vi "Populate SCL.vi"(8 "error in":errorcluster, 11 "SCL":refnum<vi>) -> (0 "error out":errorcluster, 2 "No Templates Found Message":string, 3 "At least one template file found?":bool)   [LabVIEW 2022 SP3]
doc: "Populates the SCL that displays the available VI templates and CTL templates, respectively.\n\nSCL = Single-Column Listbox"
uses:
  <vilib>/Utility/miscctls.llb/LVFontTypeDef.ctl
panel:
  out "All Template Filenames":string[](array[string])
  out "CTTs":string[](array[string])
  out "VITs":string[](array[string])
  out "VIs":string[](array[string])
  out "CTLs":string[](array[string])
  out "Templates Folder Location":path
  out "All Filenames In Folder":string[](array[string])
  # "Development\ncontrols/indicators useful for development and testing, but which are not outputs of the VI"
  # "Input\nInputs to the VI"
  # "Output\nOutputs of the VI"
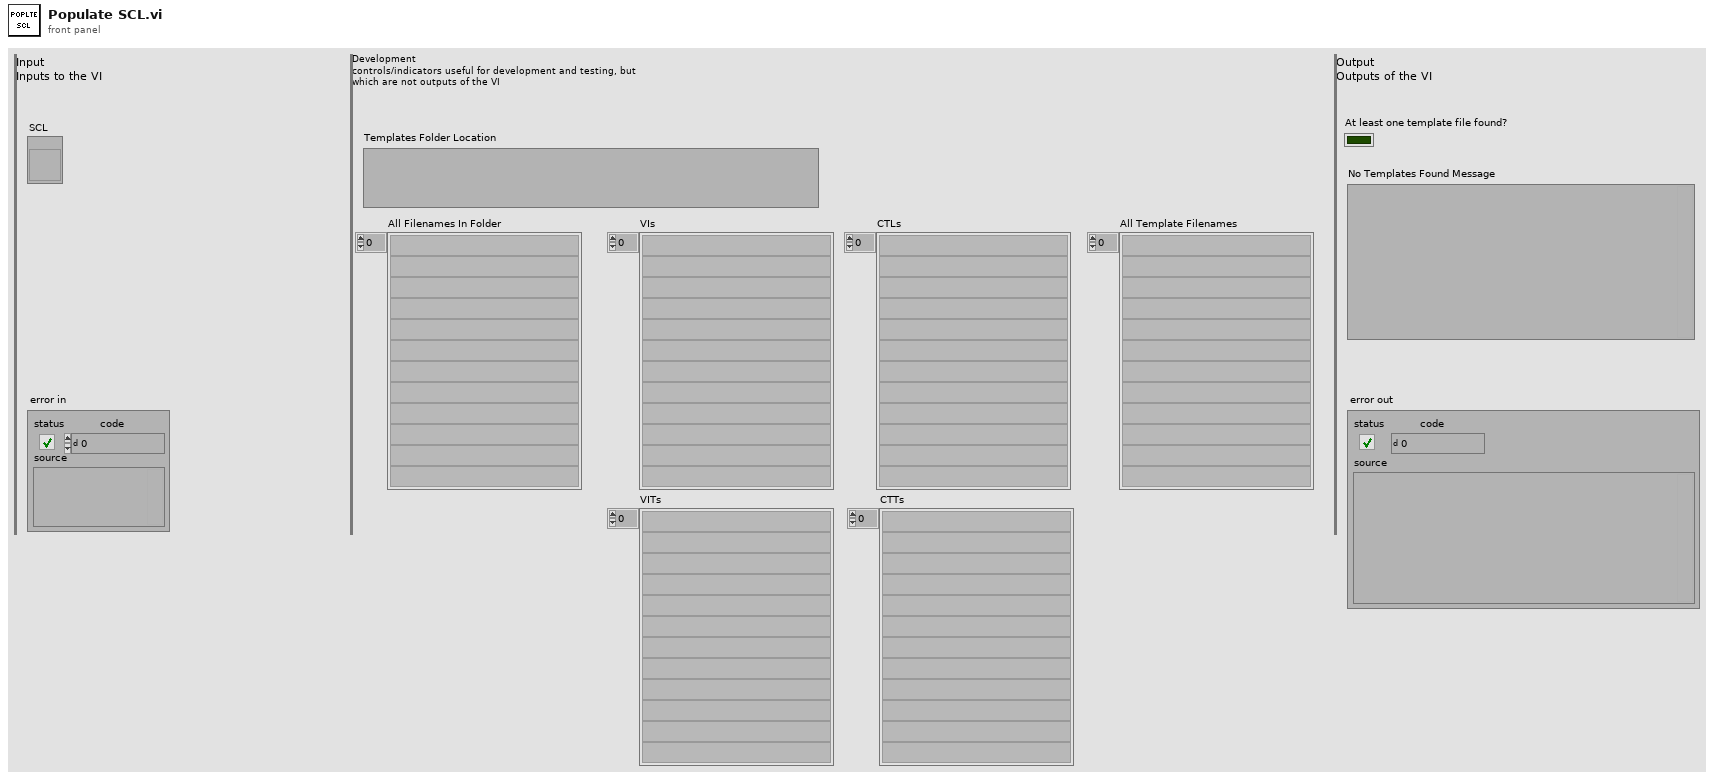
[diagram p1: front panel]
types:
  T1 = typedef "LVFontTypeDef.ctl" = cluster{"Font Name":string, "Size":u16, "Bold":bool, "Italic":bool, "Underline":bool, "Strikeout":bool, "Color":u32}
  T2 = typedef "Registry RtKey.ctl" = enum32{"HKEY_CLASSES_ROOT", "HKEY_CURRENT_USER", "HKEY_LOCAL_MACHINE", "HKEY_USERS", "HKEY_PERFORMANCE_DATA", "HKEY_CURRENT_CONFIG", "HKEY_DYN_DATA"}
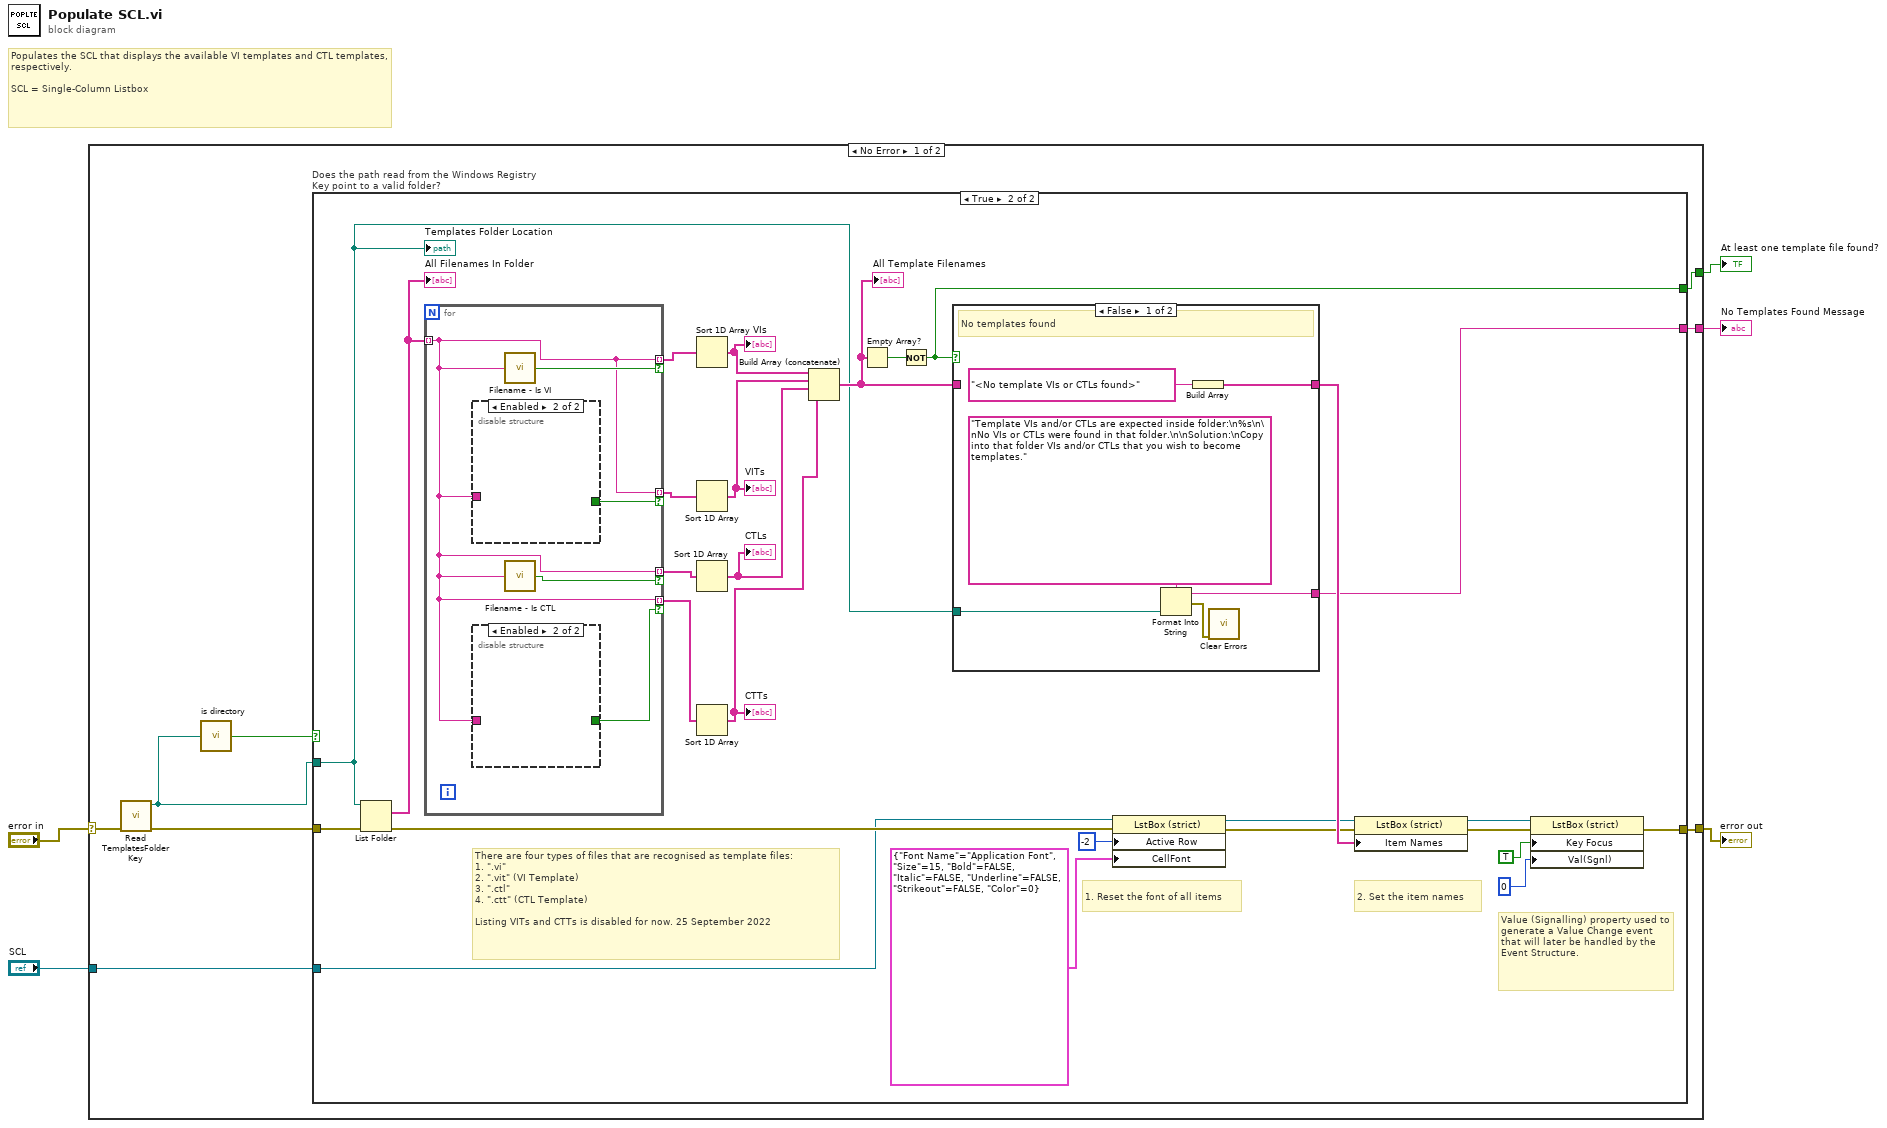
[diagram p0: block diagram]
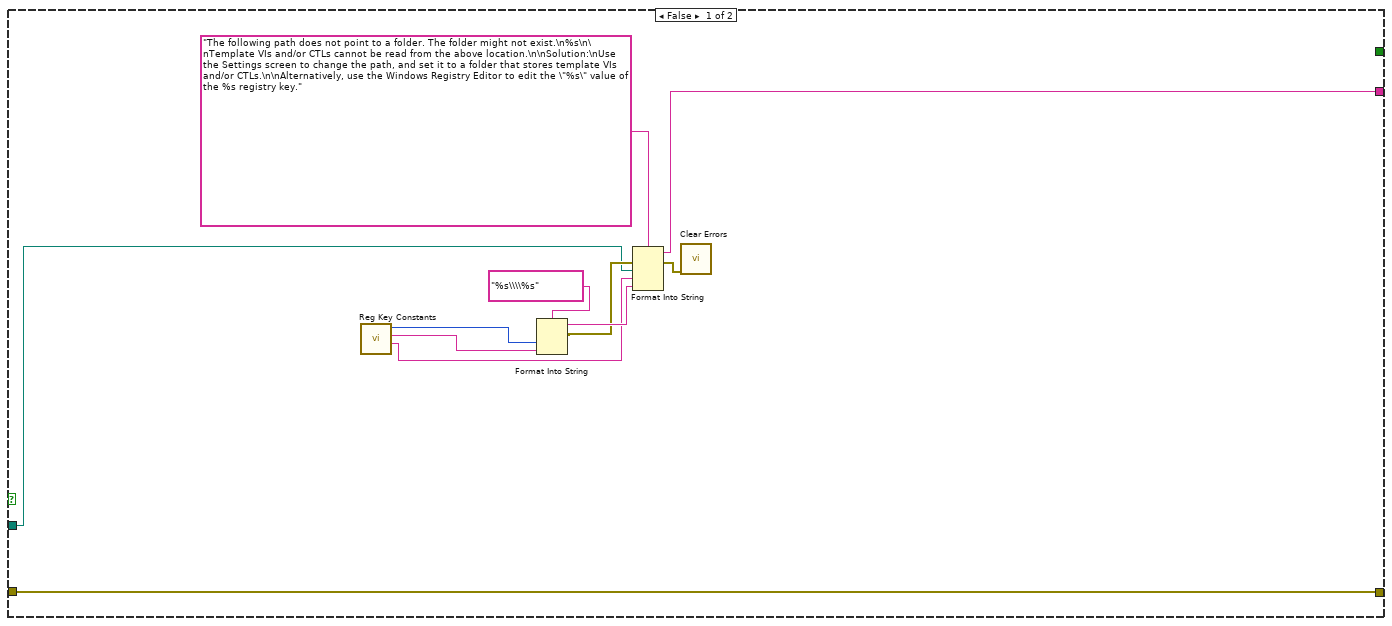
[diagram p2: hidden frame]
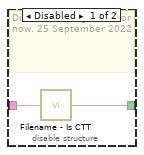
[diagram p4: hidden frame]
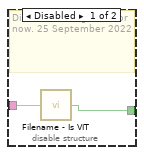
[diagram p5: hidden frame]
diagram:
  # "Populates the SCL that displays the available VI templates and CTL templates, respectively.\n\nSCL = Single-Column Listbox"
  n1 = case shown="No Error" "error in" {
    selector: "error in" -> [w10 w68]
    tunnel: [w12 w68] -> w4
    tunnel: "SCL" -> [w13 _]
    tunnel: [w11 _] -> w2
    tunnel: [w6 _] -> w1
    frame No Error {
      n2 = call "Read TemplatesFolder Key.vi"("Error In"=w10) -> ("Error Out"=w9:errorcluster, "Templates Folder Path"=w8:path)  [unwired: 9 in]
      n3 = call "is directory.vi"("Path"=w8) -> ("Does the path point to a directory (a folder)?"=w7:bool)
      n4 = case "Does the path read from the Windows Registry Key point to a valid folder?" shown="True" w7 {
        tunnel: w13 -> [_ w48]
        tunnel: [w24 w45] -> w12
        tunnel: [_ w29] -> w11
        tunnel: w9 -> [w24 w27]
        tunnel: w8 -> [w14 w26]
        tunnel: [w16 w25] -> w6
        frame False {
          n5 = call "Reg Key Constants.vi"() -> ("String Value Name"=w15:string, "Subkey Path"=w21:string, "Root Key"=w22:T2)  [unwired: 4 in, 1 out]
          n6 = Format Into String(format string="%s\\\\%s", w22, w21) -> (resulting string=w19:string, error out=w17:errorcluster)  [unwired: 2 in]
          n7 = Format Into String(format string="The following path does not point to a folder. The folder might not exist.\n%s\n\nTemplate VIs and/or CTLs cannot be read from the above location.\n\nSolution:\nUse the Settings screen to change the path, and set it to a folder that stores template VIs and/or CTLs.\n\nAlternatively, use the Windows Registry Editor to edit the \"%s\" value of the %s registry key.", error in=w17, w14, w15, w19) -> (resulting string=w16:string, error out=w18:errorcluster)  [unwired: 1 in]
          n8 = call <vilib>:"Clear Errors.vi"("error in (no error)"=w18) -> ()  [unwired: 5 in, 2 out]
        }
        frame True {
          # "Value (Signalling) property used to generate a Value Change event that will later be handled by the Event Structure."
          # "2. Set the item names"
          # "1. Reset the font of all items"
          # "There are four types of files that are recognised as template files:\n1. \".vi\"\n2. \".vit\" (VI Template)\n3. \".ctl\"\n4. \".ctt\" (CTL Template)\n\nListing VITs and CTTs is disabled for now. 25 September 2022"
          n9 = List Folder(path=w26, error in=w27) -> (filenames=w50:string[], error out=w51:errorcluster)  [unwired: 2 in, 2 out]
          "All Filenames In Folder" <- w50
          n10 = for {
            tunnel: w50 -> [w60] mode=indexing
            tunnel: [w60] -> w49 mode=indexing if=w63
            tunnel: [w60] -> w42 mode=indexing if=w62
            tunnel: [w60] -> w41 mode=indexing if=w61
            tunnel: [w60] -> w40 mode=indexing if=w59
            n11 = disable-structure shown="Enabled" {
              disable-tunnel: [w67 _] -> w62
              disable-tunnel: w60 -> [w66 _]
              frame Disabled {
                # "Disabled listing VIT's for now. 25 September 2022"
                n12 = call "Filename - Is VIT.vi"("Filename (including file extension)"=w66) -> ("Is VIT?"=w67:bool)
              }
              frame Enabled {
              }
            }
            n13 = disable-structure shown="Enabled" {
              disable-tunnel: w60 -> [w65 _]
              disable-tunnel: [w64 _] -> w59
              frame Disabled {
                # "Disabled listing CTT's for now. 25 September 2022"
                n14 = call "Filename - Is CTT.vi"("Filename (including file extension)"=w65) -> ("Is CTT?"=w64:bool)
              }
              frame Enabled {
              }
            }
            n15 = call "Filename - Is VI.vi"("Filename (including file extension)"=w60) -> ("Is VI?"=w63:bool)
            n16 = call "Filename - Is CTL.vi"("Filename (including file extension)"=w60) -> ("Is CTL?"=w61:bool)
          }
          n17 = Sort 1D Array(array=w49) -> (sorted array=w39:string[])
          "VIs" <- w39
          n18 = Sort 1D Array(array=w42) -> (sorted array=w38:string[])
          "VITs" <- w38
          n19 = Sort 1D Array(array=w41) -> (sorted array=w37:string[])
          "CTLs" <- w37
          n20 = Sort 1D Array(array=w40) -> (sorted array=w36:string[])
          "CTTs" <- w36
          n21 = Build Array (concatenate)(w39, w38, w37, w36) -> (w30:string[])
          "All Template Filenames" <- w30
          n22 = Empty Array?(array=w30) -> (empty?=w47:bool)
          n23 = Not(x=w47) -> (.not. x?=w29:bool)
          n24 = case shown="False" w29 {
            tunnel: w30 -> [_ w58]
            tunnel: [w56 w58] -> w35
            tunnel: w26 -> [w53 _]
            tunnel: [w52 _] -> w25
            frame False {
              # "No templates found"
              n25 = Format Into String(format string="Template VIs and/or CTLs are expected inside folder:\n%s\n\nNo VIs or CTLs were found in that folder.\n\nSolution:\nCopy into that folder VIs and/or CTLs that you wish to become templates.", w53) -> (resulting string=w52:string, error out=w55:errorcluster)  [unwired: 2 in]
              n26 = Build Array("<No template VIs or CTLs found>") -> (w56:string[])
              n27 = call <vilib>:"Clear Errors.vi"("error in (no error)"=w55) -> ()  [unwired: 5 in, 2 out]
            }
            frame True {
              # "One or more template files found"
            }
          }
          n28 = property class="LstBox (strict)"(reference=w48, error in=w51, "Active Row"=-2 ("Active Row:Active Row Number"), "CellFont"=T1 {"Font Name"="Application Font", "Size"=15, "Bold"=FALSE, "Italic"=FALSE, "Underline"=FALSE, "Strikeout"=FALSE, "Color"=0} ("Active Row:Cell Font")) -> (reference out=w33:refnum<vi>, error out=w32:errorcluster)
          n29 = property class="LstBox (strict)"(reference=w33, error in=w32, "Item Names"=w35) -> (reference out=w44:refnum<vi>, error out=w46:errorcluster)
          n30 = property class="LstBox (strict)"(reference=w44, error in=w46, "Key Focus"=TRUE, "Val(Sgnl)"=0 ("Value (Signaling)")) -> (error out=w45:errorcluster)  [unwired: 1 out]
          "Templates Folder Location" <- w26
        }
      }
    }
    frame Error {
    }
  }
  "error out" <- w4
  "At least one template file found?" <- w2
  "No Templates Found Message" <- w1
